vi "LPC query power.vi"(8 "error in (no error)":errorcluster, 11 "VISA resource name":refnum<visa-resource-name>="GPIB0::8::INSTR") -> (0 "error out":errorcluster, 2 "power":dbl[unit], 3 "VISA resource name out":refnum<visa-resource-name>)   [LabVIEW 2009, in "Laser Power Controller.lvclass"]
doc: "Queries the power of the LPC (laser power controller)."
uses:
  Laser Power Controller.lvclass
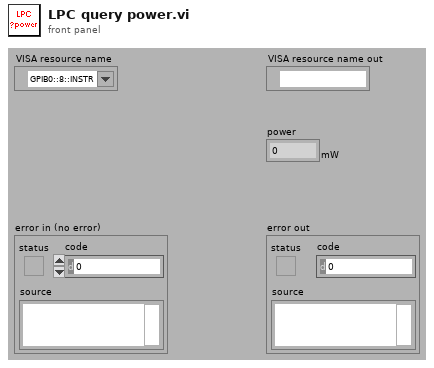
[diagram p1: front panel]
types:
  T1 = typedef "Semaphore RefNum" = refnum<k1>
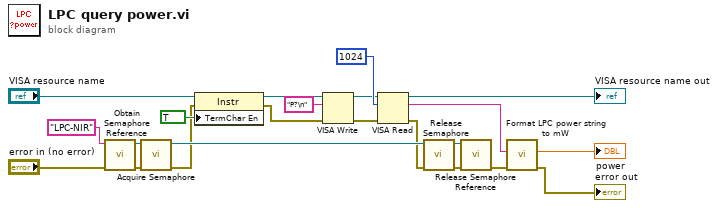
[diagram p0: block diagram]
diagram:
  n1 = call <vilib>:"Obtain Semaphore Reference.vi"("error in (no error)"="error in (no error)", "name (unnamed)"="LPC-NIR") -> ("error out"=w20:errorcluster, "semaphore"=w19:T1)  [unwired: 1 in, 3 out]
  n2 = call <vilib>:"Acquire Semaphore.vi"("error in (no error)"=w20, "semaphore"=w19) -> ("error out"=w11:errorcluster, "semaphore out"=w16:T1)  [unwired: 1 in, 3 out]
  n3 = property class="Instr"(reference="VISA resource name", error in=w11, "TermChar En"=TRUE ("Message Based Settings:Termination Character Enable")) -> (error out=w10:errorcluster)  [unwired: 1 out]
  n4 = VISA Write(VISA resource name="VISA resource name", write buffer="P?\n", error in (no error)=w10) -> (VISA resource name out=w6:refnum<visa-resource-name>, error out=w7:errorcluster)  [unwired: 1 out]
  n5 = VISA Read(VISA resource name=w6, byte count=u32 1024, error in (no error)=w7) -> (VISA resource name out=→"VISA resource name out":refnum<visa-resource-name>, read buffer=w3:string, error out=w8:errorcluster)  [unwired: 1 out]
  n6 = call <vilib>:"Release Semaphore.vi"("error in (no error)"=w8, "semaphore"=w16) -> ("error out"=w18:errorcluster, "semaphore out"=w17:T1)  [unwired: 4 out]
  n7 = call <vilib>:"Release Semaphore Reference.vi"("error in (no error)"=w18, "semaphore"=w17) -> ("error out"=w4:errorcluster)  [unwired: 9 out]
  n8 = call "Format LPC power string to mW.vi"("error in (no error)"=w4, "String"=w3) -> ("error out"=→"error out":errorcluster, "power"=→"power":dbl[unit])  [unwired: 8 out]
